vi "dds_fpga.vi"() -> ()   [LabVIEW 2018]
uses:
  <vilib>/rvi/FXPMathLib/FxpConvert/subVIs/nifxpmath_Convert_SimConfig.ctl
  <vilib>/fxp/LVFixedPointQuantizationPolicyTypeDef.ctl
  <vilib>/fxp/LVFixedPointOverflowPolicyTypeDef.ctl
  <vilib>/rvi/FXPMathLib/FxpAtan2/subVIs/nifxpmath_Atan2_SimConfig.ctl
  <vilib>/rvi/Emulation/niFpgaGetClockAttributes.vi
  <vilib>/rvi/Emulation/niFpgaSctlEmulationGetInTimedLoop.vi
  <vilib>/rvi/Emulation/niFpgaEmulationReportErrorSimple.vi
  <vilib>/rvi/Emulation/niFpgaEmulationIsFPGAContextNoSignature.vi
  <vilib>/rvi/errors/niFpgaSetErrorForExecOnDevCompSimple.vi
  <vilib>/rvi/eio/common/nirviEmuReportErrorAndStop.vi
  <vilib>/rvi/DataTransferAndStorage/Container/Common/niFpgaContainerGetUniqueNameForEmu.vi
  <vilib>/rvi/FIFO/Fifo_Resource/nirvififoEmulationSetSize.vi
  <vilib>/rvi/FIFO/Fifo_Resource/nirviFifoEmulationQueueMgr.vi
  <instcachedir>/0/nirviFifoEmulationQueueMgr_E5CAEC123FF24DC58D834DCA3CDAA9B5.lvgen/nirviFifoEmulationQueueMgr_E5CAEC123FF24DC58D834DCA3CDAA9B5_004.vi
  <vilib>/Utility/error.llb/Clear Errors.vi
  <vilib>/rvi/FIFO/Fifo_Resource/nirvififoEmulationCreateLock.vi
  <vilib>/rvi/Emulation/niFpgaProcessEmulError.vi
  <vilib>/rvi/FIFO/Fifo_Resource/nirvififoEmulationObtainLock.vi
  <vilib>/rvi/FIFO/Fifo_Resource/nirvififoEmulationReleaseLock.vi
  <vilib>/rvi/occurrence/nirviWaitOnOccurrenceBase.vi
  <vilib>/rvi/errors/nirviReportUnexpectedCaseInternalError.vi
  <vilib>/rvi/errors/nirviReportUnexpectedCaseInternalError (U32).vi
  <instcachedir>/0/nirviFifoEmulationQueueMgr_E5CAEC123FF24DC58D834DCA3CDAA9B5.lvgen/nirviFifoEmulationQueueMgr_E5CAEC123FF24DC58D834DCA3CDAA9B5_003.vi
  <vilib>/rvi/FXPMathLib/FxpConvert/simVIs/DllFxpConvertTemp_sub.vi
  <instcachedir>/0/nirviFifoEmulationQueueMgr_E5CAEC123FF24DC58D834DCA3CDAA9B5.lvgen/nirviFifoEmulationQueueMgr_E5CAEC123FF24DC58D834DCA3CDAA9B5_010.vi
  <vilib>/rvi/FIFO/Fifo_Resource/nirvififoEmulationDetermineInputValidOut.vi
  <vilib>/rvi/Emulation/niFpgaCriticalErrorInLSC.vi
  <vilib>/rvi/eio/common/nirviEmuTemplateMethod_errors.vi
  <vilib>/rvi/DataTransferAndStorage/Container/Common/niFpgaContainerExecOnDevCompGetState.vi
  <instcachedir>/0/nirviFifoEmulationQueueMgr_E5CAEC123FF24DC58D834DCA3CDAA9B5.lvgen/nirviFifoEmulationQueueMgr_E5CAEC123FF24DC58D834DCA3CDAA9B5_001.vi
  <vilib>/rvi/interface/RandomDataEmulation/niFpgaRandomDataHandleErrors.vi
  <vilib>/rvi/Memory/Memory_Emulation/niFpgaMemoryEmulationCacheClearOnFirstRun.vi
  <vilib>/rvi/Memory/Memory_Emulation/nirvimemoryEmulationManagerCache_MakeExclusive.vi
  <vilib>/rvi/Memory/Memory_Emulation/niFpgaMemoryEmulationValidateCache.vi
  <vilib>/rvi/Memory/Memory_Emulation/nirvimemoryEmulationManagerCache_InsertValue.vi
  <vilib>/rvi/Memory/Memory_Emulation/nirvimemoryEmulationManagerCache_ReleaseExclusive.vi
  <vilib>/rvi/Memory/Memory_Emulation/nirvimemoryEmulationManagerCache_GetValue.vi
  <vilib>/rvi/Memory/Memory_Emulation/nirvimemoryEmulationManagerCache_SetValue.vi
  <vilib>/rvi/Emulation/niFpgaSctlEmulationResourceMgr.vi
  <vilib>/rvi/FXPMathLib/FxpAtan2/simVIs/DllFxpAtan2Temp_sub.vi
  <vilib>/rvi/DataTransferAndStorage/Container/XNode/niFpgaContainer.xnode
  <vilib>/rvi/FIFO/Fifo_Resource/nirvififoEmulationRead.vi
  <vilib>/rvi/FXPMathLib/FxpConvert/XNode/nifxpmath_Convert.xnode
  <vilib>/rvi/FIFO/Fifo_Resource/nirvififoEmulationWrite.vi
  <vilib>/eio/EIONode/EIONode.xnode
  <vilib>/rvi/FIFO/Fifo_Resource/niFpgaFifoEmulationRefIn.vi
  <vilib>/rvi/Memory/Memory_Emulation/niFpgaMemoryEmulationRefIn.vi
  <vilib>/rvi/FXPMathLib/FxpInterpret/XNode/nifxpmath_Interpret.xnode
  <vilib>/rvi/FXPMathLib/FxpAtan2/XNode/nifxpmath_Atan2.xnode
panel:
  in  "phi_pg":fxp<+,16,0>
  in  "test_phase_mod":bool
  in  "inst_freq_offset":fxp<+/-,33,18>
  out "phi_fb_out":fxp<+/-,64,35> format="%.41g"
  out "cross_pol_phi_shifted":fxp<+/-,34,20>
  in  "phi_lower_lim":fxp<+/-,16,16>
  in  "phi_upper_lim":fxp<+/-,16,16>
  in  "phi_dc_offset":fxp<+/-,16,8>
  out "inst_freq":fxp<+/-,35,20>
  in  "phi_dg":fxp<+/-,32,16>
  in  "initialize_phase_mod":bool=TRUE
  out "sine_out_fast":i16
  out "sine out":i16
  out "phase_mod_out":fxp<+,32,0>
  in  "phase_mod_props":T1
  in  "phase_mod_scale":fxp<+,16,0>
  in  "phase_mod":bool
  in  "phi_bitshift":i16
  out "amp_lf":fxp<+,32,16>
  in  "downsample_num":i16
  out "atan2(y,x) (pi)":fxp<+/-,16,2>
  out "phi_full_out":fxp<+/-,32,18>
  out "n":i16
  in  "reset_phi":bool
  in  "discont_pos":fxp<+/-,17,3> format="%#_15g"
  in  "discont_neg":fxp<+/-,64,32>
  in  "counter_offset":u8
  out "cross_pol_amp":fxp<+,32,16>
  out "cross_pol_sig":i16
  in  "subtract_mean":bool
  out "actual_analog_in_loop_time":u32
  in  "desired_analog_in_loop_time_(uSec)":u32 caption="Count(uSec)"
  in  "custom_trig?":bool
  in  "counter_roll_over 2":u32
  in  "45_sin":bool
  in  "23_sin":bool
  in  "01_sin":bool
  in  "z_slow-dds?":bool
  in  "slow-dds_scale":fxp<+/-,16,1>
  in  "Initialize slow-dds":bool
  in  "sinewave-props_slow-dds":T1={"Frequency (periods/tick)"=0.0, "Phase offset (periods)"=0.0, "Scale factor"=0.999969482421875, "Amplitude offset"=0.0}
  in  "fast-dds_scale01":fxp<+/-,16,1>
  in  "fast-dds_scale23":fxp<+/-,16,1>
  in  "fast-dds_scale45":fxp<+/-,16,1>
  in  "sinewave-props_fast-dds":T1={"Frequency (periods/tick)"=0.0, "Phase offset (periods)"=0.0, "Scale factor"=0.999969482421875, "Amplitude offset"=0.0}
  in  "Initialize fast-dds":bool
  in  "Desired loop rate (ticks)":u32=2666666 caption="Update Interval (Ticks)"
  out "Actual loop rate":u32
  out "Sampling rate achieved?":bool
  in  "stop":bool
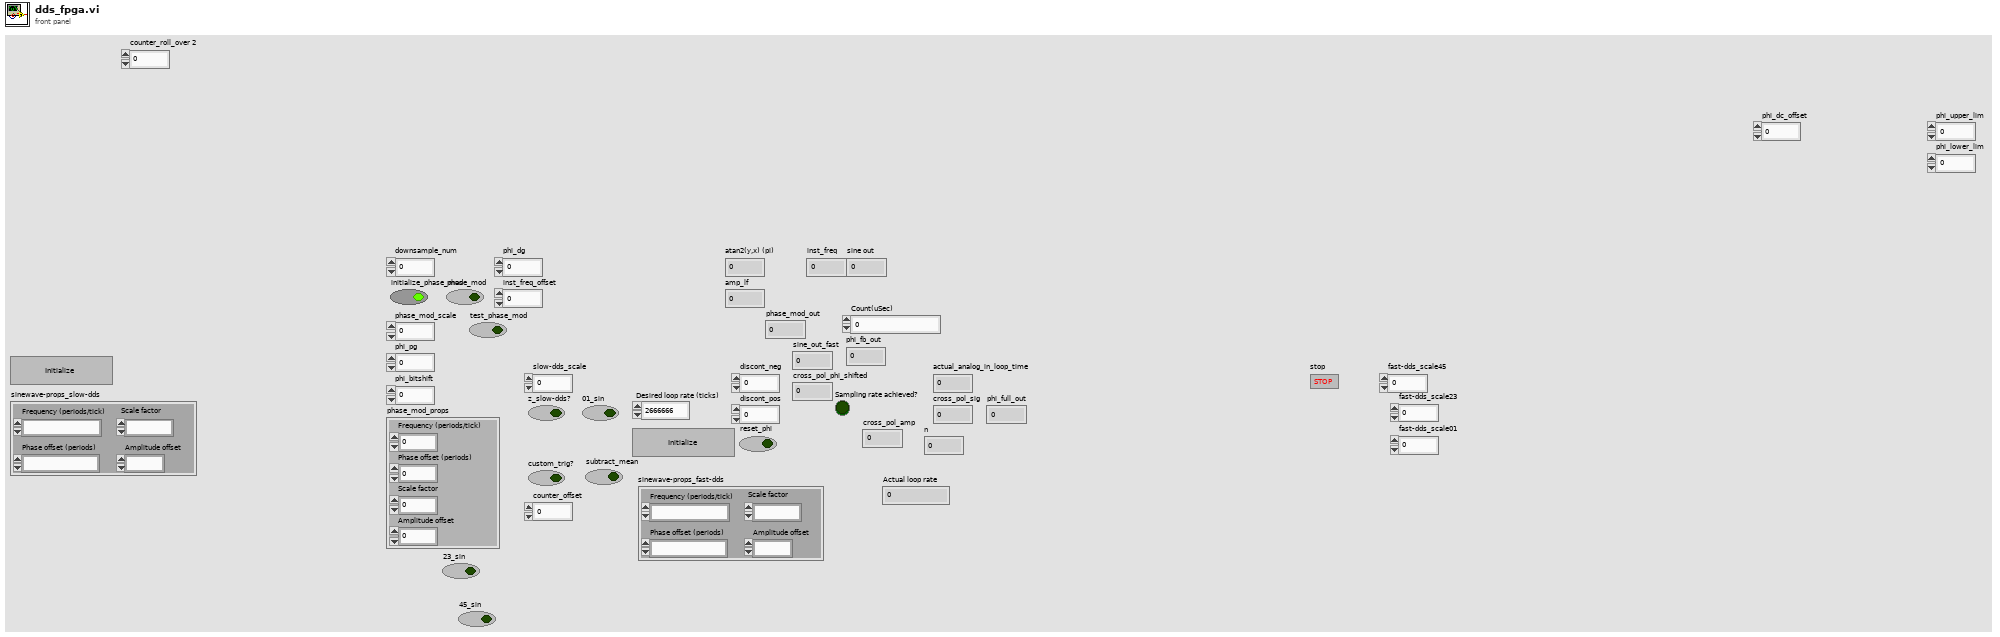
[diagram p1: front panel]
types:
  T1 = cluster{"Frequency (periods/tick)":fxp<+,32,0>, "Phase offset (periods)":fxp<+,32,0>, "Scale factor":fxp<+/-,16,1>, "Amplitude offset":fxp<+/-,16,16>}
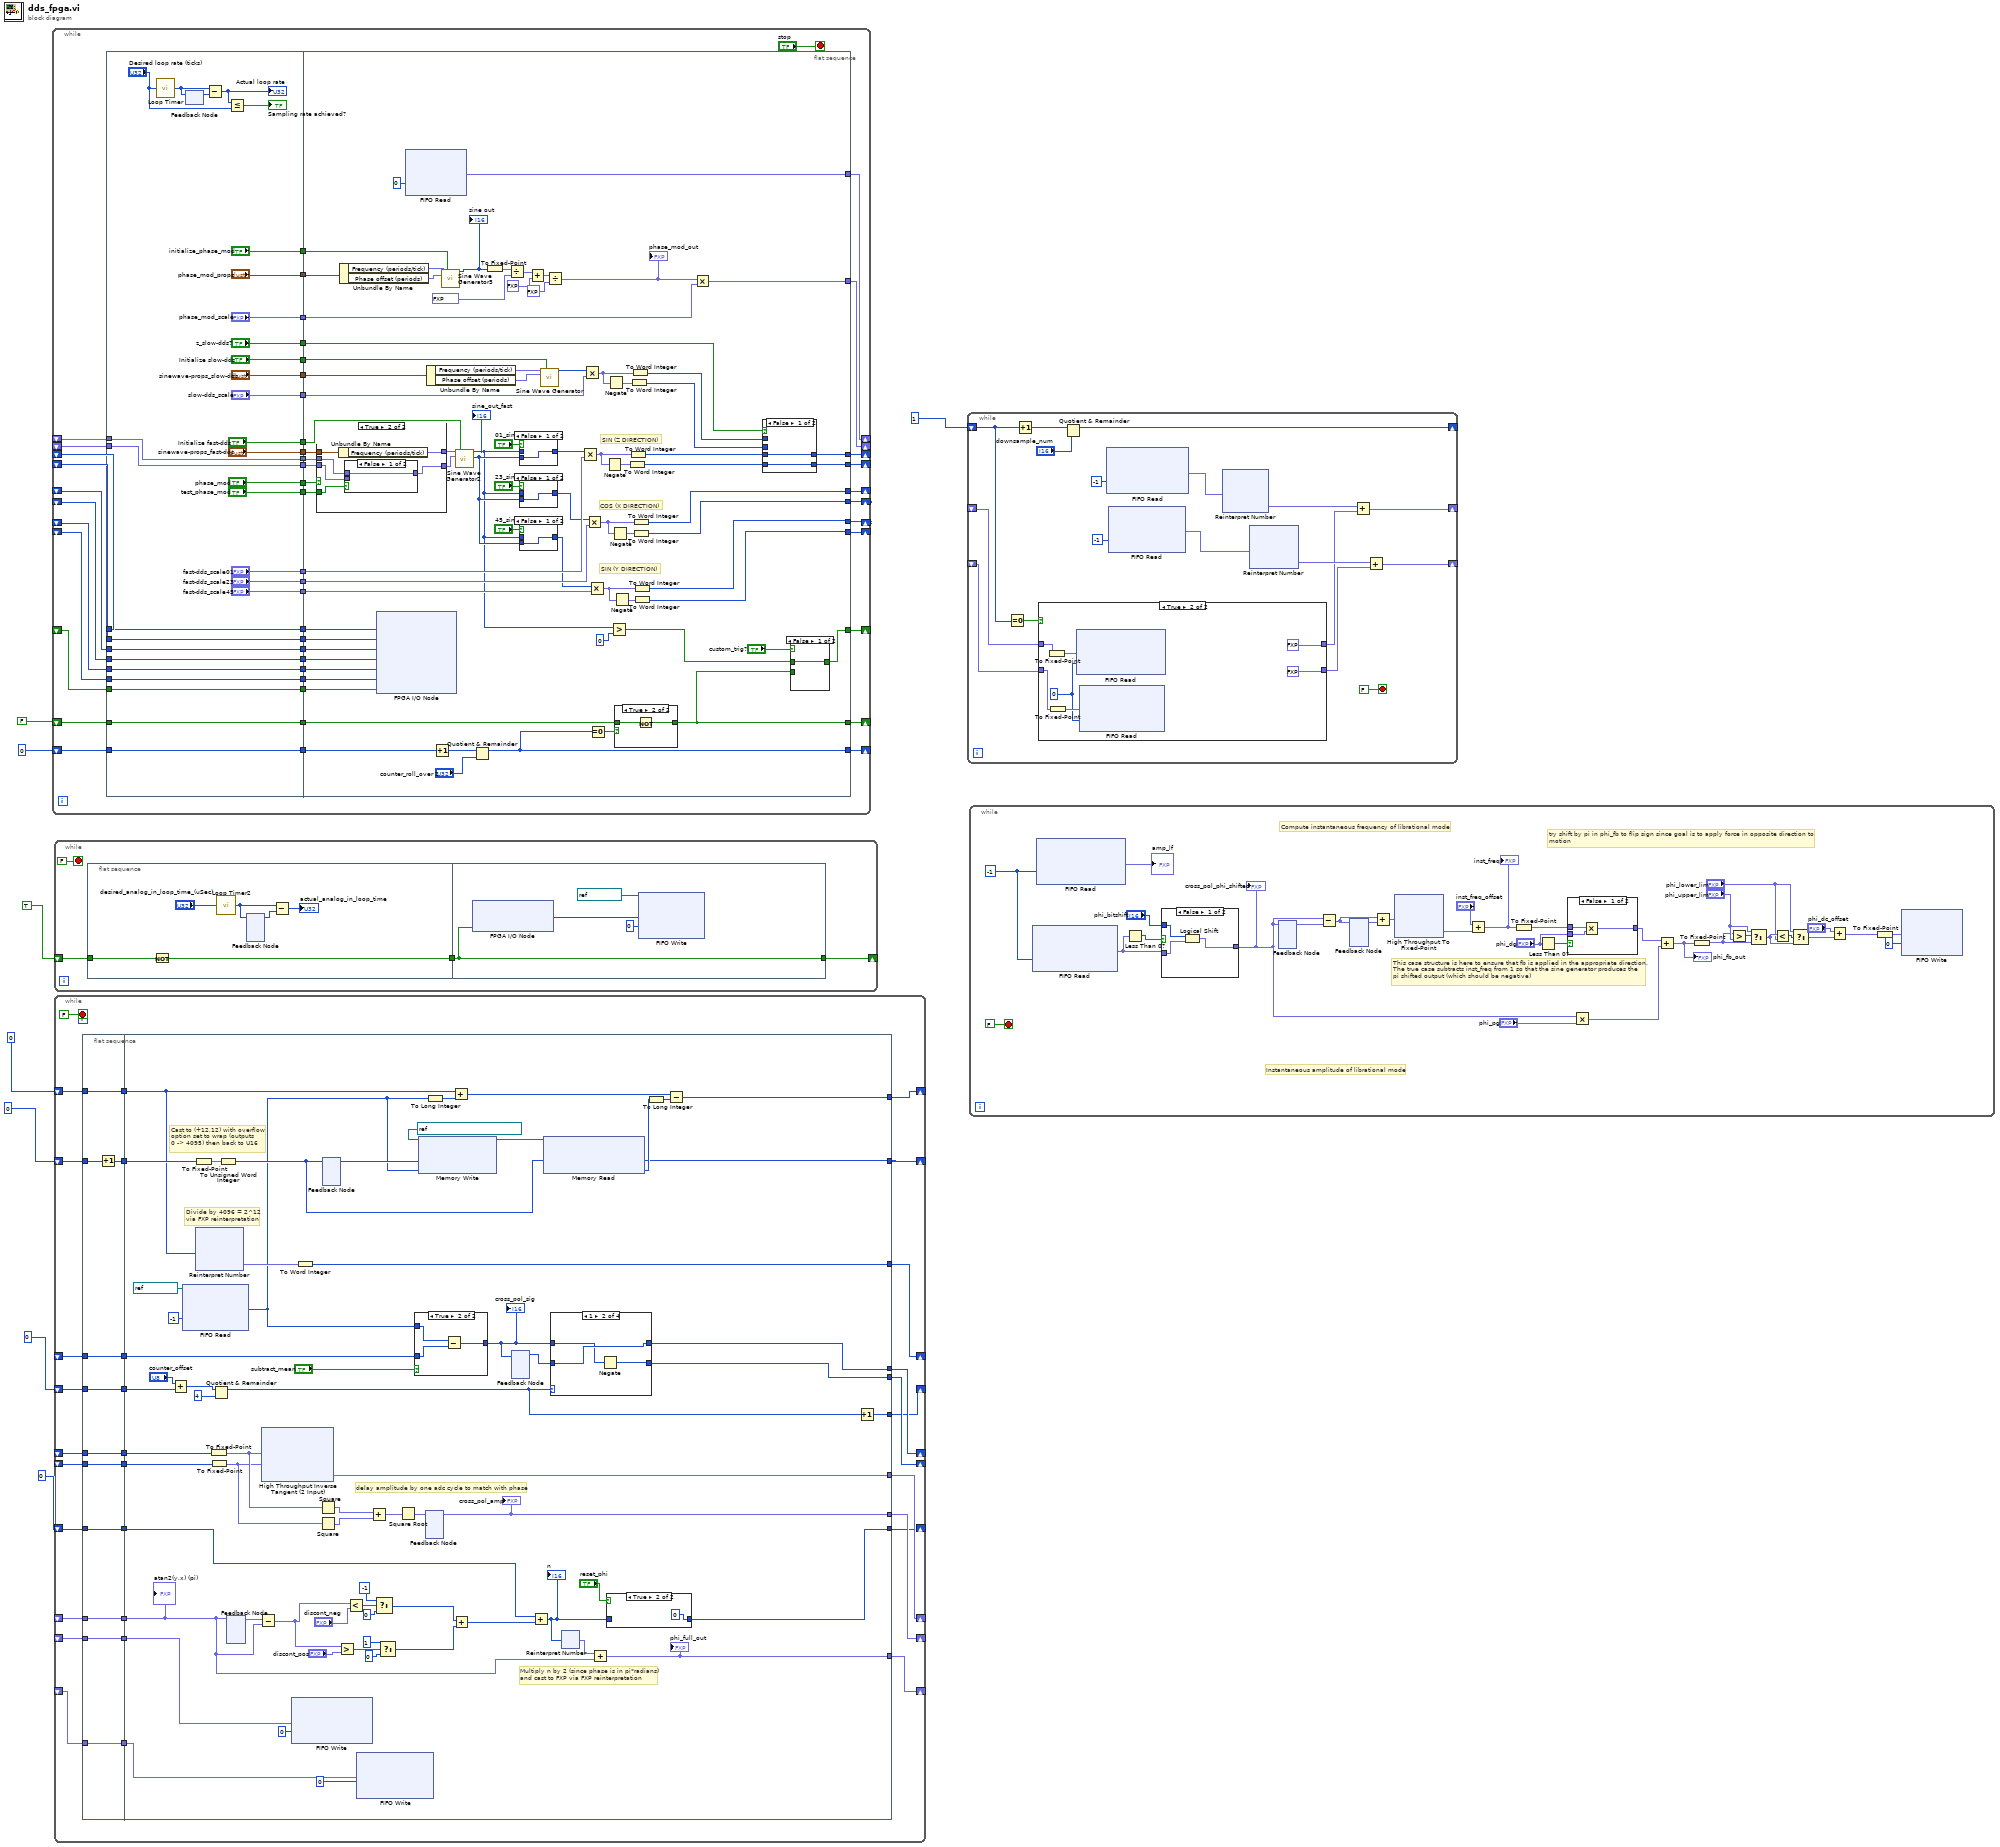
[diagram p0: block diagram]
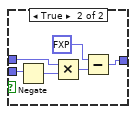
[diagram p2: hidden frame]
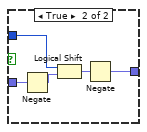
[diagram p3: hidden frame]
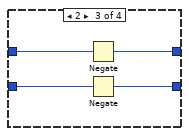
[diagram p7: hidden frame]
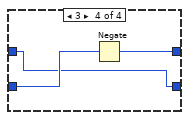
[diagram p8: hidden frame]
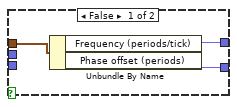
[diagram p10: hidden frame]
diagram:
  n1 = while {
    shift-right: [w20] -> _
    shift-left: _ -> [w46]
    shift-right: [w41] -> _
    shift-left: _ -> [w31]
    shift-right: [w40] -> _
    shift-left: _ -> [w28]
    shift-right: [w42] -> _
    shift-left: _ -> [w32]
    shift-right: [w43] -> _
    shift-left: _ -> [w34]
    shift-right: [w44] -> _
    shift-left: _ -> [w36]
    shift-right: [w45] -> _
    shift-left: _ -> [w38]
    shift-right: [w22] -> _
    shift-left: FALSE -> [w26]
    shift-right: [w23] -> _
    shift-left: u32 0 -> [w24]
    shift-right: [w19] -> _
    shift-left: _ -> [w17]
    shift-right: [w12] -> _
    shift-left: _ -> [w10]
    stop <- "stop" stop-if-true
    n2 = flat-sequence {
      tunnel: ["fast-dds_scale45"] -> w56
      tunnel: ["sinewave-props_fast-dds"] -> w55
      tunnel: ["Initialize fast-dds"] -> w54
      tunnel: ["fast-dds_scale23"] -> w53
      tunnel: ["fast-dds_scale01"] -> w52
      tunnel: ["sinewave-props_slow-dds"] -> w51
      tunnel: ["Initialize slow-dds"] -> w50
      tunnel: ["slow-dds_scale"] -> w49
      tunnel: ["z_slow-dds?"] -> w48
      tunnel: w46 -> [w64]
      tunnel: [w72] -> w39
      tunnel: w38 -> [w72]
      tunnel: [w71] -> w37
      tunnel: w36 -> [w71]
      tunnel: [w70] -> w35
      tunnel: w34 -> [w70]
      tunnel: [w69] -> w33
      tunnel: w32 -> [w69]
      tunnel: w31 -> [w68]
      tunnel: [w68] -> w30
      tunnel: [w67] -> w29
      tunnel: w28 -> [w67]
      tunnel: [w66] -> w27
      tunnel: w26 -> [w66]
      tunnel: [w65] -> w25
      tunnel: w24 -> [w65]
      tunnel: [w64] -> w21
      tunnel: [w63] -> w18
      tunnel: w17 -> [w63]
      tunnel: ["phase_mod"] -> w16
      tunnel: ["phase_mod_scale"] -> w15
      tunnel: ["phase_mod_props"] -> w14
      tunnel: ["initialize_phase_mod"] -> w13
      tunnel: [w58] -> w11
      tunnel: w10 -> [w58]
      tunnel: ["test_phase_mod"] -> w9
      tunnel: w56 -> [w157]
      tunnel: w55 -> [w156]
      tunnel: w54 -> [w108]
      tunnel: w53 -> [w155]
      tunnel: w52 -> [w154]
      tunnel: w51 -> [w151]
      tunnel: w50 -> [w152]
      tunnel: w49 -> [w146]
      tunnel: w48 -> [w140]
      tunnel: [w131] -> w45
      tunnel: [w130] -> w44
      tunnel: [w112] -> w43
      tunnel: [w111] -> w42
      tunnel: [w110] -> w41
      tunnel: [w109] -> w40
      tunnel: w39 -> [w129]
      tunnel: w37 -> [w128]
      tunnel: w35 -> [w127]
      tunnel: w33 -> [w126]
      tunnel: w30 -> [w125]
      tunnel: w29 -> [w124]
      tunnel: w27 -> [w120]
      tunnel: w25 -> [w119]
      tunnel: [w118] -> w23
      tunnel: [w114] -> w22
      tunnel: w21 -> [w117]
      tunnel: [w116] -> w20
      tunnel: [w104] -> w19
      tunnel: w18 -> [w88]
      tunnel: w16 -> [w106]
      tunnel: w15 -> [w105]
      tunnel: w14 -> [w101]
      tunnel: w13 -> [w93]
      tunnel: [w90] -> w12
      tunnel: w11 -> [w89]
      tunnel: w9 -> [w87]
      frame #0 {
        n3 = call "Loop Timer"("Count(Ticks)"="Desired loop rate (ticks)") -> ("Tick Count(Ticks)"=w83:u32)
        n4 = feedback-in #1(w83) -> ()
        n5 = feedback #1() -> (w82:u32)  [unwired: 1 out]
        n6 = Subtract(x=w83, y=w82) -> (x-y=w86:u32)
        "Actual loop rate" <- w86
        n7 = Less Or Equal?(x=w86, y="Desired loop rate (ticks)") -> (x <= y?=→"Sampling rate achieved?":bool)
      }
      frame #1 {
        # "SIN (Y DIRECTION)"
        # "COS (X DIRECTION)"
        # "SIN (Z DIRECTION)"
        n8 = case shown="True" w106 {
          tunnel: [w167 w172] -> w164
          tunnel: w156 -> [w166 w173]
          tunnel: [w165 w170] -> w107
          tunnel: w89 -> [_ w171]
          tunnel: w88 -> [_ w169]
          tunnel: w87 -> [_ w168]
          frame False {
            n9 = Unbundle By Name(w166) -> ("Frequency (periods/tick)"=w167:fxp<+,32,0>, "Phase offset (periods)"=w165:fxp<+,32,0>)
          }
          frame True {
            n10 = Unbundle By Name(w173) -> ("Frequency (periods/tick)"=w172:fxp<+,32,0>)
            n11 = case shown="False" w168 {
              tunnel: w171 -> [w174 _]
              tunnel: [w174 w175] -> w170
              tunnel: w169 -> [_ w175]
              frame False {
              }
              frame True {
              }
            }
          }
        }
        n12 = Unbundle By Name(w101) -> ("Frequency (periods/tick)"=w103:fxp<+,32,0>, "Phase offset (periods)"=w102:fxp<+,32,0>)
        n13 = xnode "FPGA I/O Node"("Connector0/AO0"=w129, "Connector0/AO1"=w128, "Connector0/AO2"=w127, "Connector0/AO3"=w126, "Connector0/AO4"=w125, "Connector0/AO5"=w124, "Connector0/DIO0"=w117) -> ()  [unwired: 7 in, 7 out]
        n14 = xnode ("FIFO Read")("Timeout"=0) -> ("Element"=w90:fxp<+,32,0>)  [unwired: 1 in, 2 out]
        n15 = Unbundle By Name(w151) -> ("Frequency (periods/tick)"=w150:fxp<+,32,0>, "Phase offset (periods)"=w149:fxp<+,32,0>)
        n16 = Increment(x=w119) -> (x+1=w123:u32)
        n17 = call "Sine Wave Generator3"("frequency (periods/tick)"=w103, "reset"=w93, "phase offset (periods)"=w102) -> ("sine out"=w92:i16)  [unwired: 12 in]
        "sine out" <- w92
        n18 = call "Sine Wave Generator2"("frequency (periods/tick)"=w164, "reset"=w108, "phase offset (periods)"=w107) -> ("sine out"=w134:i16, "cosine out"=w135:i16)  [unwired: 11 in]
        "sine_out_fast" <- w134
        n19 = Quotient & Remainder(x=w123, y="counter_roll_over 2") -> (x-y*floor(x/y)=w118:u32)  [unwired: 1 out]
        n20 = To Fixed-Point(number=w92) -> (fixed-point=w100:fxp<+/-,32,16>)  [unwired: 1 in]
        n21 = Divide(x=w100, y=fxp<+,16,15> 32767.5) -> (x/y=w98:fxp<+/-,32,16>)
        n22 = case shown="False" "01_sin" {
          tunnel: w134 -> [_ w186]
          tunnel: w135 -> [w185 _]
          tunnel: [w185 w186] -> w138
          frame False {
          }
          frame True {
          }
        }
        n23 = case shown="False" "23_sin" {
          tunnel: w134 -> [_ w184]
          tunnel: w135 -> [w183 _]
          tunnel: [w183 w184] -> w133
          frame False {
          }
          frame True {
          }
        }
        n24 = case shown="False" "45_sin" {
          tunnel: w134 -> [_ w182]
          tunnel: w135 -> [w181 _]
          tunnel: [w181 w182] -> w132
          frame False {
          }
          frame True {
          }
        }
        n25 = Add(x=w98, y=fxp<+,1,1> 1.0 ("x")) -> (x+y=w96:fxp<+,32,2>)
        n26 = call "Sine Wave Generator"("frequency (periods/tick)"=w150, "reset"=w152, "phase offset (periods)"=w149) -> ("sine out"=w145:i16)  [unwired: 12 in]
        n27 = Divide(x=w96, y=fxp<+,1,2> 2.0) -> (x/y=w94:fxp<+,32,0>)
        "phase_mod_out" <- w94
        n28 = Multiply(x=w138, y=w154) -> (x*y=w163:fxp<+/-,32,17>)
        n29 = Multiply(x=w145, y=w146) -> (x*y=w148:fxp<+/-,32,17>)
        n30 = Multiply(x=w133, y=w155) -> (x*y=w160:fxp<+/-,32,17>)
        n31 = Multiply(x=w132, y=w157) -> (x*y=w158:fxp<+/-,32,17>)
        n32 = Equal To 0?(x=w118) -> (x = 0?=w121:bool)
        n33 = Negate(x=w163) -> (-x=w162:fxp<+/-,31,16>)
        n34 = Negate(x=w148) -> (-x=w147:fxp<+/-,31,16>)
        n35 = Greater?(x=w134, y=i16 0) -> (0:w115:bool)
        n36 = Negate(x=w160) -> (-x=w161:fxp<+/-,31,16>)
        n37 = Negate(x=w158) -> (-x=w159:fxp<+/-,31,16>)
        n38 = case shown="True" w121 {
          tunnel: w120 -> [w178 w180]
          tunnel: [w178 w179] -> w114
          frame False {
          }
          frame True {
            n39 = Not(x=w180) -> (.not. x?=w179:bool)
          }
        }
        n40 = To Word Integer(number=w162) -> (16bit integer=w144:i16)
        n41 = To Word Integer(number=w163) -> (16bit integer=w143:i16)
        n42 = To Word Integer(number=w147) -> (16bit integer=w142:i16)
        n43 = To Word Integer(number=w148) -> (16bit integer=w141:i16)
        n44 = To Word Integer(number=w160) -> (16bit integer=w112:i16)
        n45 = To Word Integer(number=w161) -> (16bit integer=w111:i16)
        n46 = To Word Integer(number=w158) -> (16bit integer=w110:i16)
        n47 = To Word Integer(number=w159) -> (16bit integer=w109:i16)
        n48 = Multiply(x=w94, y=w105) -> (x*y=w104:fxp<+,32,0>)
        n49 = case shown="False" w140 {
          tunnel: [w188 w190] -> w130
          tunnel: w144 -> [w188 _]
          tunnel: [w187 w189] -> w131
          tunnel: w143 -> [w187 _]
          tunnel: w142 -> [_ w190]
          tunnel: w141 -> [_ w189]
          frame False {
          }
          frame True {
          }
        }
        n50 = case shown="False" "custom_trig?" {
          tunnel: [w176 w177] -> w116
          tunnel: w115 -> [w176 _]
          tunnel: w114 -> [_ w177]
          frame False {
          }
          frame True {
          }
        }
      }
    }
  }
  n51 = while {
    shift-right: [w191] -> _
    shift-left: TRUE -> [w193]
    stop <- FALSE stop-if-true
    n52 = flat-sequence {
      tunnel: w193 -> [w196]
      tunnel: [w195] -> w192
      tunnel: w192 -> [w201]
      tunnel: [w201] -> w191
      frame #0 {
        n53 = Not(x=w196) -> (.not. x?=w195:bool)
        n54 = call "Loop Timer2"("Count(uSec)"="desired_analog_in_loop_time_(uSec)") -> ("Tick Count(uSec)"=w199:u32)
        n55 = feedback-in #2(w199) -> ()
        n56 = feedback #2() -> (w198:u32)  [unwired: 1 in]
        n57 = Subtract(x=w199, y=w198) -> (x-y=→"actual_analog_in_loop_time":u32)
      }
      frame #1 {
        n58 = xnode "FPGA I/O Node"("Connector0/DIO1"=w201) -> ("Connector0/AI0"=w203:i16)  [unwired: 2 in, 2 out]
        n59 = xnode ("FIFO Write")("Element"=w203, "Timeout"=0, "FIFO In"=refnum<k21> "acq_data") -> ()  [unwired: 2 out]
      }
    }
  }
  n60 = while {
    shift-right: [w234] -> _
    shift-left: 0 -> [w233]
    shift-right: [w231] -> _
    shift-left: u16 0 -> [w230]
    shift-right: [w229] -> _
    shift-left: _ -> [w228]
    shift-right: [w224] -> _
    shift-left: _ -> [w221]
    shift-right: [w223] -> _
    shift-left: _ -> [w220]
    shift-right: [w218] -> _
    shift-left: _ -> [w212]
    shift-right: [w217] -> _
    shift-left: _ -> [w216]
    shift-right: [w213] -> _
    shift-left: _ -> [w209]
    shift-right: [w206] -> _
    shift-left: i16 0 -> [w207]
    shift-right: [w205] -> _
    shift-left: u8 0 -> [w226]
    stop <- FALSE stop-if-true
    n61 = flat-sequence {
      tunnel: w233 -> [w246]
      tunnel: [w246] -> w235
      tunnel: w230 -> [w245]
      tunnel: [w244] -> w232
      tunnel: w228 -> [w243]
      tunnel: [w243] -> w227
      tunnel: w226 -> [w242]
      tunnel: [w242] -> w225
      tunnel: [w241] -> w222
      tunnel: w221 -> [w241]
      tunnel: w220 -> [w240]
      tunnel: [w240] -> w219
      tunnel: w216 -> [w239]
      tunnel: [w239] -> w215
      tunnel: [w236] -> w214
      tunnel: w212 -> [w238]
      tunnel: [w238] -> w211
      tunnel: [w237] -> w210
      tunnel: w209 -> [w237]
      tunnel: w207 -> [w236]
      tunnel: w235 -> [w298]
      tunnel: [w305] -> w234
      tunnel: w232 -> [w302]
      tunnel: [w299] -> w231
      tunnel: [w296] -> w229
      tunnel: w227 -> [w291]
      tunnel: w225 -> [w276]
      tunnel: [w287] -> w224
      tunnel: [w286] -> w223
      tunnel: w222 -> [w285]
      tunnel: w219 -> [w284]
      tunnel: [w279] -> w218
      tunnel: [w278] -> w217
      tunnel: w215 -> [w258]
      tunnel: w214 -> [w261]
      tunnel: [w257] -> w213
      tunnel: w211 -> [w256]
      tunnel: w210 -> [w253]
      tunnel: [w250] -> w206
      tunnel: [w248] -> w205
      frame #0 {
        n62 = Increment(x=w245) -> (x+1=w244:u16)
      }
      frame #1 {
        # "Multiply n by 2 (since phase is in pi*radians)\nand cast to FXP via FXP reinterpretation"
        # "Cast to (+12,12) with overflow\noption set to wrap (outputs \n0 -> 4095) then back to U16"
        # "Divide by 4096 = 2^12 \nvia FXP reinterpretation"
        # "delay amplitude by one adc cycle to match with phase"
        n63 = Add(x="counter_offset", y=w276) -> (x+y=w275:u8)
        n64 = xnode ("FIFO Read")("Timeout"=-1, "FIFO In"=refnum<k21> "acq_data") -> ("Element"=w292:i16)  [unwired: 2 out]
        n65 = To Fixed-Point(number=w302) -> (fixed-point=w301:fxp<+,12,12>)  [unwired: 1 in]
        n66 = xnode "Reinterpret Number"("x"=w298) -> ("y"=w297:fxp<+/-,32,20>)
        n67 = To Fixed-Point(number=w285) -> (fixed-point=w283:fxp<+/-,16,16>)  [unwired: 1 in]
        n68 = To Fixed-Point(number=w284) -> (fixed-point=w282:fxp<+/-,16,16>)  [unwired: 1 in]
        n69 = Quotient & Remainder(x=w275, y=u8 4) -> (x-y*floor(x/y)=w247:u8)  [unwired: 1 out]
        n70 = To Unsigned Word Integer(number=w301) -> (unsigned 16bit integer=w299:u16)
        n71 = feedback-in #3(w258) -> ()
        n72 = feedback #3() -> (w273:fxp<+/-,16,2>)  [unwired: 1 in]
        n73 = Subtract(x=w273, y=w258) -> (x-y=w249:fxp<+/-,17,3>)
        n74 = xnode "High Throughput Inverse Tangent (2 Input)"("y"=w283, "x"=w282) -> ("atan2(y,x) (pi)"=w278:fxp<+/-,16,2>)
        n75 = xnode ("FIFO Write")("Element"=w256, "Timeout"=0) -> ()  [unwired: 1 in, 2 out]
        n76 = To Word Integer(number=w297) -> (16bit integer=w296:i16)
        n77 = Square(x=w283) -> (x^2=w281:fxp<+,31,31>)
        n78 = Square(x=w282) -> (x^2=w280:fxp<+,31,31>)
        n79 = feedback-in #4(w299) -> ()
        n80 = feedback #4() -> (w300:u16)  [unwired: 1 in]
        n81 = Greater?(x=w249, y="discont_pos") -> (0:w268:bool)
        n82 = Less?(x=w249, y="discont_neg") -> (x < y?=w272:bool)
        n83 = xnode ("FIFO Write")("Element"=w253, "Timeout"=0) -> ()  [unwired: 1 in, 2 out]
        n84 = Add(x=w281, y=w280) -> (x+y=w255:fxp<+,32,32>)
        n85 = Select(t=i16 -1, s=w272, f=i16 0) -> (s? t:f=w265:i16)
        n86 = Select(t=i16 1, s=w268, f=i16 0) -> (s? t:f=w264:i16)
        n87 = Square Root(x=w255) -> (sqrt(x)=w254:fxp<+,32,16>)
        n88 = case shown="True" "subtract_mean" {
          tunnel: w292 -> [w352 w355]
          tunnel: w291 -> [_ w354]
          tunnel: [w352 w353] -> w289
          frame False {
          }
          frame True {
            n89 = Subtract(x=w355, y=w354) -> (x-y=w353:i16)
          }
        }
        "cross_pol_sig" <- w289
        n90 = xnode ("Memory Write")("Address"=w300, "Data"=w292, "Memory In"=refnum<k21> "cross_pol_light_moving_avg") -> ("Memory Out"=w307:refnum<k21>)
        n91 = feedback-in #5(w254) -> ()
        n92 = feedback #5() -> (w279:fxp<+,32,16>)  [unwired: 1 in]
        "cross_pol_amp" <- w279
        n93 = To Long Integer(number=w292) -> (32bit integer=w309:i32)
        n94 = Add(x=w298, y=w309) -> (x+y=w306:i32)
        n95 = Add(x=w265, y=w264) -> (x+y=w263:i16)
        n96 = feedback-in #6(w289) -> ()
        n97 = feedback #6() -> (w288:i16)  [unwired: 1 in]
        n98 = Add(x=w261, y=w263) -> (x+y=w260:i16)
        "n" <- w260
        n99 = xnode ("Memory Read")("Address"=w299, "Memory In"=w307) -> ("Data"=w303:i16)  [unwired: 1 out]
        n100 = case shown="1" w247 {
          tunnel: w289 -> [w341 w342 w348 w349]
          tunnel: w288 -> [w340 w344 w345 w351]
          tunnel: [w341 w344 w347 w350] -> w287
          tunnel: [w340 w343 w346 w349] -> w286
          frame 0, Default {
          }
          frame 1 {
            n101 = Negate(x=w342) -> (-x=w343:i16)
          }
          frame 2 {
            n102 = Negate(x=w348) -> (-x=w347:i16)
            n103 = Negate(x=w345) -> (-x=w346:i16)
          }
          frame 3 {
            n104 = Negate(x=w351) -> (-x=w350:i16)
          }
        }
        n105 = xnode "Reinterpret Number"("x"=w260) -> ("y"=w259:fxp<+/-,16,17>)
        n106 = Add(x=w259, y=w258) -> (x+y=w257:fxp<+/-,32,18>)
        "phi_full_out" <- w257
        n107 = case shown="True" "reset_phi" {
          tunnel: w260 -> [w310 _]
          tunnel: [w310 i16 0] -> w250
          frame False {
          }
          frame True {
          }
        }
        n108 = To Long Integer(number=w303) -> (32bit integer=w304:i32)
        n109 = Subtract(x=w306, y=w304) -> (x-y=w305:i32)
        n110 = Increment(x=w247) -> (x+1=w248:u8)
        "atan2(y,x) (pi)" <- w258
      }
    }
  }
  n111 = while {
    shift-right: [w367] -> _
    shift-left: i16 1 -> [w365]
    shift-right: [w361] -> _
    shift-left: _ -> [w360]
    shift-right: [w363] -> _
    shift-left: _ -> [w359]
    stop <- FALSE stop-if-true
    n112 = Equal To 0?(x=w365) -> (x = 0?=w366:bool)
    n113 = Increment(x=w365) -> (x+1=w369:i16)
    n114 = case shown="True" w366 {
      tunnel: w360 -> [w374 w378]
      tunnel: w359 -> [w375 w381]
      tunnel: [w375 fxp<+,64,32> 0.0] -> w358
      tunnel: [w374 fxp<+/-,64,32> 0.0] -> w357
      frame False {
      }
      frame True {
        w376 = 0
        n115 = To Fixed-Point(number=w381) -> (fixed-point=w382:fxp<+,32,16>)  [unwired: 1 in]
        n116 = To Fixed-Point(number=w378) -> (fixed-point=w377:fxp<+/-,32,18>)  [unwired: 1 in]
        n117 = xnode ("FIFO Read")("Element"=w382, "Timeout"=w376) -> ()  [unwired: 1 in, 2 out]
        n118 = xnode ("FIFO Read")("Element"=w377, "Timeout"=w376) -> ()  [unwired: 1 in, 2 out]
      }
    }
    n119 = Quotient & Remainder(x=w369, y="downsample_num") -> (x-y*floor(x/y)=w367:i16)  [unwired: 1 out]
    n120 = xnode ("FIFO Read")("Timeout"=-1) -> ("Element"=w371:fxp<+,32,16>)  [unwired: 1 in, 2 out]
    n121 = xnode ("FIFO Read")("Timeout"=-1) -> ("Element"=w370:fxp<+/-,32,18>)  [unwired: 1 in, 2 out]
    n122 = xnode "Reinterpret Number"("x"=w371) -> ("y"=w364:fxp<+/-,32,9>)
    n123 = xnode "Reinterpret Number"("x"=w370) -> ("y"=w362:fxp<+/-,32,9>)
    n124 = Add(x=w364, y=w358) -> (x+y=w363:fxp<+,64,32>)
    n125 = Add(x=w362, y=w357) -> (x+y=w361:fxp<+/-,64,32>)
  }
  n126 = while {
    stop <- FALSE stop-if-true
    w414 = -1 ("Timeout")
    # "This case structure is here to ensure that fb is applied in the appropriate direction.\nThe true case subtracts inst_freq from 1 so that the sine generator produces the \npi shifted output (which should be negative)"
    # "try shift by pi in phi_fb to flip sign since goal is to apply force in opposite direction to \nmotion"
    # "Instantaneous amplitude of librational mode"
    # "Compute instantaneous frequency of librational mode"
    n127 = xnode ("FIFO Read")("Timeout"=w414) -> ("Element"=w410:fxp<+/-,32,18>)  [unwired: 1 in, 2 out]
    n128 = xnode ("FIFO Read")("Timeout"=w414) -> ("Element"=→"amp_lf":fxp<+,32,16>)  [unwired: 1 in, 2 out]
    n129 = Less Than 0?(x=w410) -> (x < 0?=w411:bool)
    n130 = case shown="False" w411 {
      tunnel: w410 -> [w447 w453]
      tunnel: "phi_bitshift" -> [w448 w452]
      tunnel: [w446 w449] -> w385
      frame False {
        n131 = Logical Shift(y=w448, x=w447) -> (x << y=w446:fxp<+/-,32,18>)
      }
      frame True {
        n132 = Negate(x=w453) -> (-x=w451:fxp<+/-,32,18>)
        n133 = Logical Shift(y=w452, x=w451) -> (x << y=w450:fxp<+/-,32,18>)
        n134 = Negate(x=w450) -> (-x=w449:fxp<+/-,32,18>)
      }
    }
    "cross_pol_phi_shifted" <- w385
    n135 = feedback-in #7(w385) -> ()
    n136 = feedback #7() -> (w408:fxp<+/-,32,18>)  [unwired: 1 in]
    n137 = Subtract(x=w385, y=w408) -> (x-y=w406:fxp<+/-,32,18>)
    n138 = feedback #8() -> (w407:fxp<+/-,32,18>)  [unwired: 1 in]
    n139 = feedback-in #8(w406) -> ()
    n140 = Add(x=w406, y=w407) -> (x+y=w405:fxp<+/-,33,19>)
    n141 = xnode "High Throughput To Fixed-Point"("x"=w405) -> ("y"=w395:fxp<+/-,33,18>)
    n142 = Add(x="inst_freq_offset", y=w395) -> (x+y=w393:fxp<+/-,34,19>)
    "inst_freq" <- w393
    n143 = To Fixed-Point(number=w393) -> (fixed-point=w390:fxp<+/-,32,18>)  [unwired: 1 in]
    n144 = Less Than 0?(x="phi_dg") -> (x < 0?=w392:bool)
    n145 = case shown="False" w392 {
      tunnel: "phi_dg" -> [w416 w423]
      tunnel: w390 -> [w417 w421]
      tunnel: [w415 w418] -> w387
      frame False {
        n146 = Multiply(x=w417, y=w416) -> (x*y=w415:fxp<+/-,64,34>)
      }
      frame True {
        n147 = Negate(x=w423) -> (-x=w422:fxp<+/-,33,17>)
        n148 = Multiply(x=w421, y=w422) -> (x*y=w420:fxp<+/-,63,33>)
        n149 = Subtract(x=fxp<+/-,63,33> 1.0, y=w420) -> (x-y=w418:fxp<+/-,64,34>)
      }
    }
    n150 = Multiply(x=w385, y="phi_pg") -> (x*y=w383:fxp<+/-,48,18>)
    n151 = Add(x=w387, y=w383) -> (x+y=w386:fxp<+/-,64,35>)
    "phi_fb_out" <- w386
    n152 = To Fixed-Point(number=w386) -> (fixed-point=w389:fxp<+/-,64,35>)  [unwired: 1 in]
    n153 = Greater?(x=w389, y="phi_upper_lim") -> (0:w403:bool)
    n154 = Select(t="phi_upper_lim", s=w403, f=w389) -> (s? t:f=w401:fxp<+/-,64,35>)
    n155 = Less?(x=w401, y="phi_lower_lim") -> (x < y?=w402:bool)
    n156 = Select(t="phi_lower_lim", s=w402, f=w401) -> (s? t:f=w400:fxp<+/-,64,35>)
    n157 = Add(x="phi_dc_offset", y=w400) -> (x+y=w388:fxp<+/-,64,36>)
    n158 = To Fixed-Point(number=w388) -> (fixed-point=w397:fxp<+,32,0>)  [unwired: 1 in]
    n159 = xnode ("FIFO Write")("Element"=w397, "Timeout"=0) -> ()  [unwired: 1 in, 2 out]
  }
